vi "cvII_01_01.vi"() -> ()   [LabVIEW 2013]
uses:
  <vilib>/measure/NI_MABase.lvlib
  <vilib>/Waveform/WDTOps.llb/WDT Append Waveforms DBL.vi
  <vilib>/measure/NI_MAPro.lvlib
  <vilib>/measure/maspectr.llb/FFT Power Spectrum and PSD for 1 Chan.vi
panel:
  in  "stop":bool
  in  "Averaging parameters":T1
  out "Power Spectrum":cluster{"f0":dbl, "df":dbl, "magnitude":dbl[]}(graph)
  out "Time Waveform":waveform(dbl)(graph)
  in  "Sampling Info":cluster{"Fs":dbl, "#s":dbl} {"Fs" format="%#.2p"}
  in  "Noise Amplitude":dbl(slide) scale=0.0..10.0
  in  "Sine Amplitude":dbl(slide) scale=0.0..10.0
  in  "Sine Frequency":dbl(slide) scale=0.0..500.0
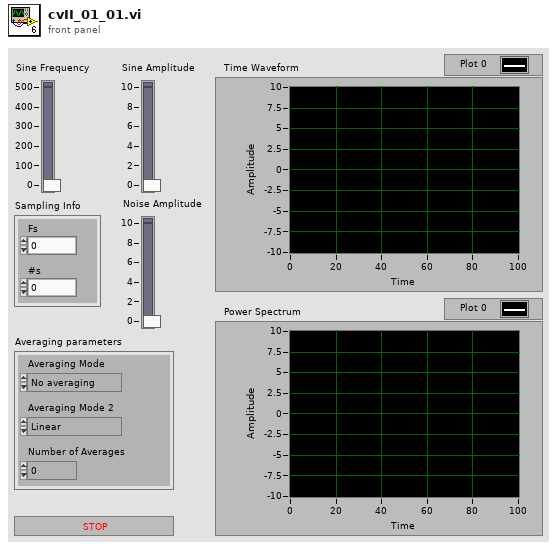
[diagram p1: front panel]
types:
  T1 = cluster{"Averaging Mode":enum16{"No averaging", "Vector averaging", "RMS averaging", "Peak hold"}, "Averaging Mode 2":enum16{"Linear", "Exponential"}, "Number of Averages":dbl}
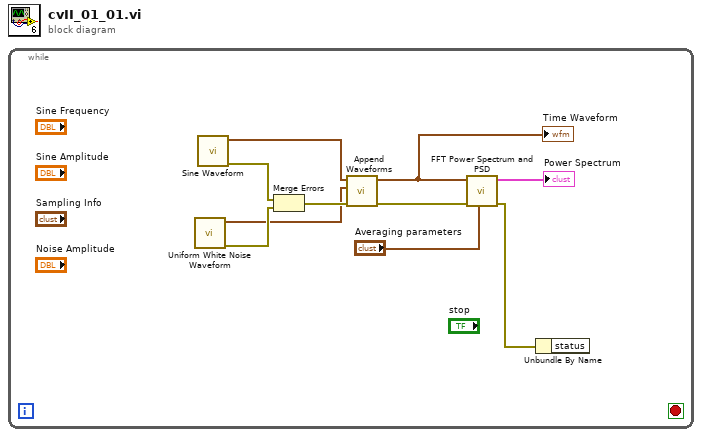
[diagram p0: block diagram]
diagram:
  n1 = while {
    stop <- _ stop-if-true
    n2 = call <vilib>:"Uniform White Noise Waveform.vi"() -> ("error out"=w8:errorcluster, "signal out"=w4:waveform(dbl))  [unwired: 10 in]
    n3 = call <vilib>:"Sine Waveform.vi"() -> ("error out"=w7:errorcluster, "signal out"=w6:waveform(dbl))  [unwired: 10 in]
    n4 = Merge Errors(w7, w8) -> (w5:errorcluster)
    n5 = call-poly <vilib>:"Append Waveforms.vi"("error in (no error)"=w5, "waveform B"=w4, "waveform A"=w6) -> ("error out"=w3:errorcluster, "waveform out"=w2:waveform(dbl))  [unwired: 7 in]
    "Time Waveform" <- w2
    n6 = call-poly <vilib>:"FFT Power Spectrum and PSD.vi"("averaging parameters"="Averaging parameters", "error in (no error)"=w3, "time signal"=w2) -> ("error out"=w10:errorcluster, "Power Spectrum / PSD"=→"Power Spectrum":cluster{"f0":dbl, "df":dbl, "magnitude":dbl[]})  [unwired: 5 in, 2 out]
    n7 = Unbundle By Name(w10) -> ()  [unwired: 1 out]
  }
